vi "IMUprocess live readings.vi"(6 "Acc sensivity":dbl=8192.0 format="%#_13g", 8 "Gyro sensivity":dbl=131.072 format="%#_13g", 9 "Bias":T1, 10 "Sensor Data in":u16[](array[numeric]), 11 "error in (no error)":errorcluster) -> (0 "Gyro deg/s":cluster{dbl, dbl, dbl}, 1 "Accel g's":cluster{dbl, dbl, dbl}, 3 "error out":errorcluster)   [LabVIEW 2016]
doc: "Inputs\nRaw data from MPU9250\nBias\nAccelerometer sensivity\nGyroscope sensivity\n\nOutputs\nAccelerometer readings\nGyroscope readings\n\nThis VI process the raw data from the IMU, first it bitshifts the data, then it removes the bias from the readings and finally it divdes the data with the sensivity (Which can be found in the data sheet and depends on how the registers are set up)"
panel:
  # "8192"
  # "2048"
  # "16.4"
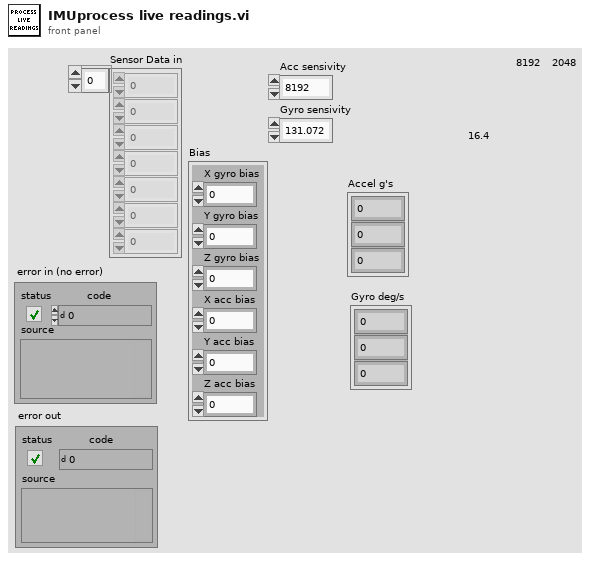
[diagram p1: front panel]
types:
  T1 = cluster{"X gyro bias":dbl, "Y gyro bias":dbl, "Z gyro bias":dbl, "X acc bias":dbl, "Y acc bias":dbl, "Z acc bias":dbl}
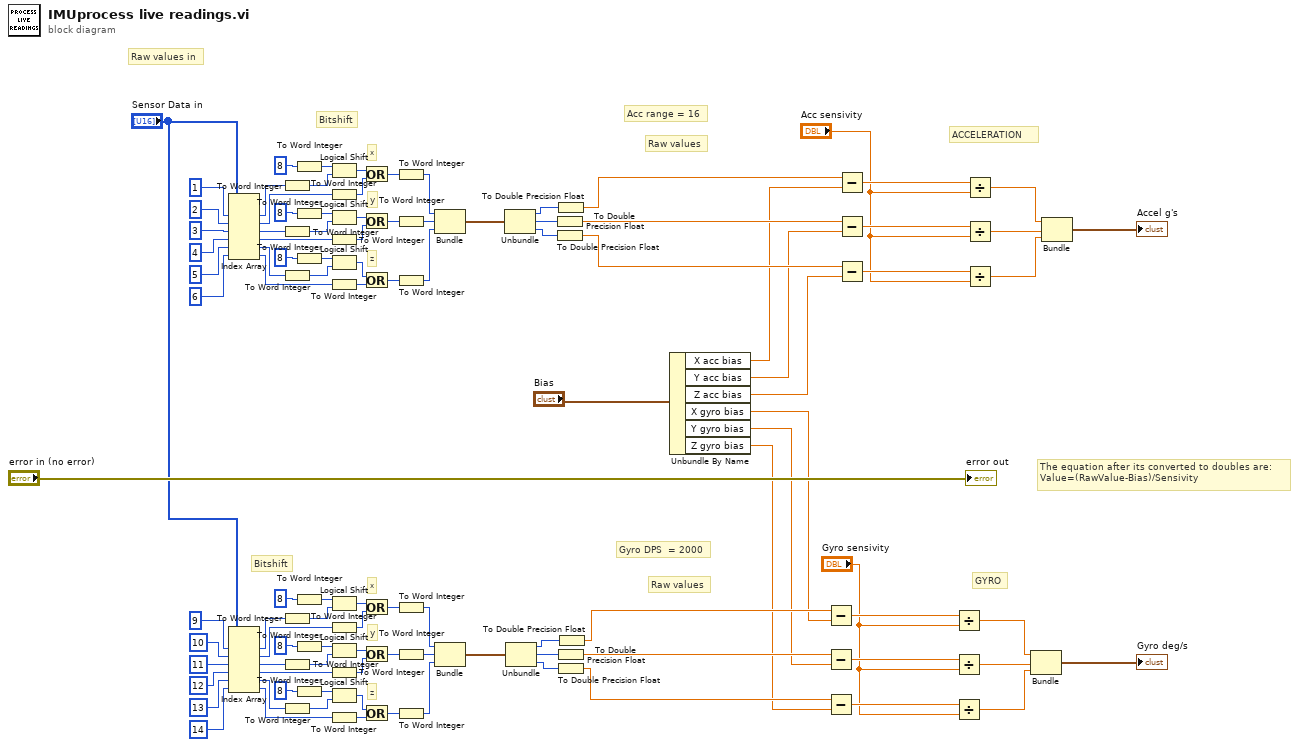
[diagram p0: block diagram]
diagram:
  # "Raw values in"
  # "The equation after its converted to doubles are:\nValue=(RawValue-Bias)/Sensivity"
  # "Raw values"
  # "Raw values"
  # "Bitshift"
  # "Bitshift"
  # "GYRO"
  # "ACCELERATION"
  # "Acc range = 16"
  # "Gyro DPS  = 2000"
  # "z"
  # "y"
  # "x"
  # "z"
  # "y"
  # "x"
  n1 = Index Array(array="Sensor Data in", index #1=1 ("index"), index #2=2 ("index"), index #3=3 ("index"), index #4=4 ("index"), index #5=5 ("index"), index #6=6 ("index")) -> (element #1=w82:u16, element #2=w77:u16, element #3=w69:u16, element #4=w65:u16, element #5=w60:u16, element #6=w59:u16)
  n2 = Index Array(array="Sensor Data in", index #1=9 ("index"), index #2=10 ("index"), index #3=11 ("index"), index #4=12 ("index"), index #5=13 ("index"), index #6=14 ("index")) -> (element #1=w39:u16, element #2=w38:u16, element #3=w37:u16, element #4=w36:u16, element #5=w35:u16, element #6=w34:u16)
  n3 = To Word Integer(number=w82) -> (16bit integer=w81:i16)
  n4 = To Word Integer(number=w69) -> (16bit integer=w66:i16)
  n5 = To Word Integer(number=w60) -> (16bit integer=w61:i16)
  n6 = To Word Integer(number=w39) -> (16bit integer=w46:i16)
  n7 = To Word Integer(number=w37) -> (16bit integer=w52:i16)
  n8 = To Word Integer(number=w35) -> (16bit integer=w56:i16)
  n9 = To Word Integer(number=i16 8 ("y")) -> (16bit integer=w80:i16)
  n10 = To Word Integer(number=i16 8 ("y")) -> (16bit integer=w67:i16)
  n11 = To Word Integer(number=i16 8 ("y")) -> (16bit integer=w62:i16)
  n12 = To Word Integer(number=i16 8 ("y")) -> (16bit integer=w47:i16)
  n13 = To Word Integer(number=i16 8 ("y")) -> (16bit integer=w51:i16)
  n14 = To Word Integer(number=i16 8 ("y")) -> (16bit integer=w55:i16)
  n15 = Logical Shift(y=w80, x=w81) -> (x << y=w99:i16)
  n16 = To Word Integer(number=w77) -> (16bit integer=w78:i16)
  n17 = Logical Shift(y=w67, x=w66) -> (x << y=w98:i16)
  n18 = To Word Integer(number=w65) -> (16bit integer=w64:i16)
  n19 = Logical Shift(y=w62, x=w61) -> (x << y=w97:i16)
  n20 = To Word Integer(number=w59) -> (16bit integer=w58:i16)
  n21 = Logical Shift(y=w47, x=w46) -> (x << y=w40:i16)
  n22 = To Word Integer(number=w38) -> (16bit integer=w49:i16)
  n23 = Logical Shift(y=w51, x=w52) -> (x << y=w41:i16)
  n24 = To Word Integer(number=w36) -> (16bit integer=w53:i16)
  n25 = Logical Shift(y=w55, x=w56) -> (x << y=w42:i16)
  n26 = To Word Integer(number=w34) -> (16bit integer=w57:i16)
  n27 = Or(x=w99, y=w78) -> (x .or. y?=w88:i16)
  n28 = Or(x=w98, y=w64) -> (x .or. y?=w84:i16)
  n29 = Or(x=w97, y=w58) -> (x .or. y?=w85:i16)
  n30 = Or(x=w40, y=w49) -> (x .or. y?=w43:i16)
  n31 = Or(x=w41, y=w53) -> (x .or. y?=w45:i16)
  n32 = Or(x=w42, y=w57) -> (x .or. y?=w44:i16)
  n33 = To Word Integer(number=w88) -> (16bit integer=w87:i16)
  n34 = To Word Integer(number=w84) -> (16bit integer=w86:i16)
  n35 = To Word Integer(number=w85) -> (16bit integer=w83:i16)
  n36 = To Word Integer(number=w43) -> (16bit integer=w33:i16)
  n37 = To Word Integer(number=w45) -> (16bit integer=w32:i16)
  n38 = To Word Integer(number=w44) -> (16bit integer=w31:i16)
  n39 = Bundle(w87, w86, w83) -> (w89:cluster{i16, i16, i16})  [unwired: 1 in]
  n40 = Bundle(w33, w32, w31) -> (w70:cluster{i16, i16, i16})  [unwired: 1 in]
  n41 = Unbundle(w89) -> (w76:i16, w75:i16, w74:i16)
  n42 = Unbundle(w70) -> (w71:i16, w72:i16, w73:i16)
  n43 = To Double Precision Float(number=w75) -> (double precision float=w5:dbl)
  n44 = To Double Precision Float(number=w74) -> (double precision float=w6:dbl)
  n45 = To Double Precision Float(number=w76) -> (double precision float=w7:dbl)
  n46 = To Double Precision Float(number=w72) -> (double precision float=w28:dbl)
  n47 = To Double Precision Float(number=w73) -> (double precision float=w27:dbl)
  n48 = To Double Precision Float(number=w71) -> (double precision float=w29:dbl)
  n49 = Unbundle By Name("Bias") -> ("X acc bias"=w4:dbl, "Y acc bias"=w3:dbl, "Z acc bias"=w2:dbl, "X gyro bias"=w18:dbl, "Y gyro bias"=w17:dbl, "Z gyro bias"=w16:dbl)
  n50 = Subtract(x=w29, y=w18) -> (x-y=w26:dbl)
  n51 = Subtract(x=w28, y=w17) -> (x-y=w25:dbl)
  n52 = Subtract(x=w27, y=w16) -> (x-y=w24:dbl)
  n53 = Subtract(x=w7, y=w4) -> (x-y=w15:dbl)
  n54 = Subtract(x=w5, y=w3) -> (x-y=w14:dbl)
  n55 = Subtract(x=w6, y=w2) -> (x-y=w13:dbl)
  n56 = Divide(x=w26, y="Gyro sensivity") -> (x/y=w22:dbl)
  n57 = Divide(x=w25, y="Gyro sensivity") -> (x/y=w21:dbl)
  n58 = Divide(x=w24, y="Gyro sensivity") -> (x/y=w20:dbl)
  n59 = Divide(x=w15, y="Acc sensivity") -> (x/y=w12:dbl)
  n60 = Divide(x=w14, y="Acc sensivity") -> (x/y=w11:dbl)
  n61 = Divide(x=w13, y="Acc sensivity") -> (x/y=w10:dbl)
  n62 = Bundle(w22, w21, w20) -> (→"Gyro deg/s":cluster{dbl, dbl, dbl})  [unwired: 1 in]
  n63 = Bundle(w12, w11, w10) -> (→"Accel g's":cluster{dbl, dbl, dbl})  [unwired: 1 in]
  "error out" <- "error in (no error)"
